vi "Imaign Pulse Control.vi"() -> ()   [LabVIEW 2012]
doc: "This VI is an example of how to use subVIs from the QC 9000 series driver to programmatically configure multiple channels and the system timer (To). This VI initializes the pulse generator, gets the number of channels in the unit, configures individual channel(s), configures the system timer (To), initiate pulse generation, and then closes communications with the pulse generator. By default the VI DOES NOT stop pulse generation when exiting!!! Not all trigger and gate features are supported by all models covered by this driver. Selection of an unsupported function will generate a software error and the command is not sent to the hardware.\n\n\nNotes:\n1) The pulse generator keypad is returned to \"Local\" mode when this VI terminates in order to restore manual control to the user.\n2) VISA Version 3.3 or higher must be installed to use this instrument driver."
uses:
  Examples/Support/Channel Parameters.ctl
  Examples/Support/System Parameters.ctl
  Quantum Composers 9000 Series.lvlib
panel:
  in  "VISA resource":refnum<visa-resource-name>="GPIB0::4::INSTR"
  in  "System Paramaters":T1={"Sys Period"=0.02, "Sys Mode"=enum."Single", "Sys Burst #"=0, "Sys DC On"=10, "Sys DC Off"=20, "Sys State"=TRUE, "Sys Gate"=TRUE, "Sys Trig Edge"=TRUE, "Sys Ext Mode"=enum."Triggered", "Sys Trig Lev"=2.0, "Sys Gate Lev "=2.5, "Sys Gate Mode"=enum."Disabled"} {"Sys Gate Lev" format="%.4p"; "Sys Trig Lev" format="%.4p"; "Sys Period" format="%.6p"}
  in  "Channel Parameters":T2[](array[typedef])=[{"Channel"=1, "Chan State"=TRUE, "Chan Sync Source"=0, "Chan Gate Logic"=enum."Disabled", "Chan Mode"=enum."Normal", "Chan Wait #"=0, "Chan Delay"=0.0, "Chan Width"=1e-05, "Chan Burst #"=0, "Chan DC On"=0, "Chan DC Off"=0, "Chan Polarity"=FALSE, "Chan MUX Value"=3, "Chan Level Out"=enum."TTL", "Chan Lev Adjust"=5.0, "Chan Gate Mode"=enum."Disabled"}, {"Channel"=2, "Chan State"=TRUE, "Chan Sync Source"=0, "Chan Gate Logic"=enum."Disabled", "Chan Mode"=enum."Normal", "Chan Wait #"=0, "Chan Delay"=0.0105, "Chan Width"=1e-05, "Chan Burst #"=0, "Chan DC On"=0, "Chan DC Off"=0, "Chan Polarity"=FALSE, "Chan MUX Value"=-1, "Chan Level Out"=enum."TTL", "Chan Lev Adjust"=0.0, "Chan Gate Mode"=enum."Disabled"}, {"Channel"=3, "Chan State"=TRUE, "Chan Sync Source"=0, "Chan Gate Logic"=enum."Disabled", "Chan Mode"=enum."Normal", "Chan Wait #"=30, "Chan Delay"=0.03, "Chan Width"=0.03, "Chan Burst #"=30, "Chan DC On"=30, "Chan DC Off"=30, "Chan Polarity"=FALSE, "Chan MUX Value"=-1, "Chan Level Out"=enum."TTL", "Chan Lev Adjust"=0.0, "Chan Gate Mode"=enum."Disabled"}, {"Channel"=4, "Chan State"=TRUE, "Chan Sync Source"=0, "Chan Gate Logic"=enum."Disabled", "Chan Mode"=enum."Normal", "Chan Wait #"=40, "Chan Delay"=0.04, "Chan Width"=0.04, "Chan Burst #"=40, "Chan DC On"=40, "Chan DC Off"=40, "Chan Polarity"=FALSE, "Chan MUX Value"=-1, "Chan Level Out"=enum."TTL", "Chan Lev Adjust"=0.0, "Chan Gate Mode"=enum."Disabled"}] {"Chan Sync Source" items=["System (To)", "Channel A", "Channel B", "Channel C", "Channel D", "Channel E", "Channel F", "Channel G", "Channel H"]; "Chan Width" format="%.3p"; "Chan Delay" format="%.3p"; "Chan MUX Value" min=-1 max=255; "Chan Lev Adjust" min=0.0 max=5.0 format="%.3p"; "Channel" items=["Channel A"=1, "Channel B"=2, "Channel C"=3, "Channel D"=4, "Channel E"=5, "Channel F"=6, "Channel G"=7, "Channel H"=8]}
  # "9000 Series\nPulse Generator\nExample Program"
  # "Notes:\n1.  The channel parameters \"Burst #\", \"DC On\", \"DC Off\", and \"Adjustable\" are only updated when operating in the corresponding mode.\n2.  The system parameters  \"Burst #\", \"DC On\", \"DC Off\", and \"Trig Level\"` are only updated when operating in the corresponding mode."
  # "Input"
  # "Triggered"
  # "Gated"
  # "Mode"
  # "Burst"
  # "Duty\nCycle"
  # "Input"
  # "Normal\nSingle\nBurst"
  # "Burst"
  # "Duty Cycle"
  # "Output"
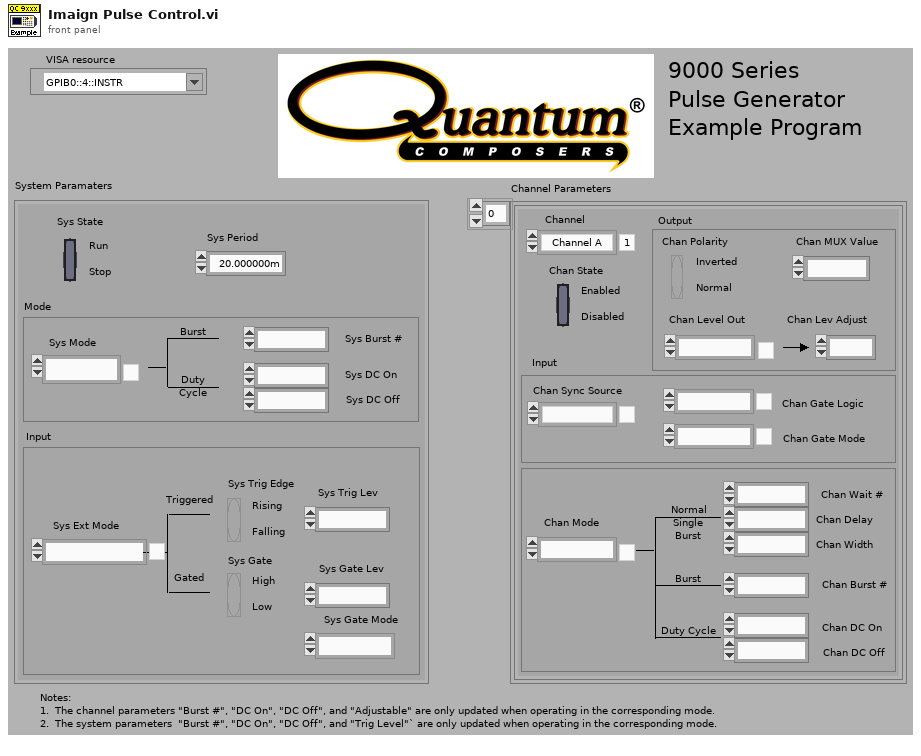
[diagram p1: front panel]
types:
  T1 = typedef "System Parameters.ctl" = cluster{"Sys Period":dbl, "Sys Mode":enum16{"Normal", "Single", "Burst", "Duty Cycle"}, "Sys Burst #":i32, "Sys DC On":i32, "Sys DC Off":i32, "Sys State":bool, "Sys Gate":bool, "Sys Trig Edge":bool, "Sys Ext Mode":enum16{"Disabled", "Triggered", "Gated", "Triggered & Gated"}, "Sys Trig Lev":dbl, "Sys Gate Lev ":dbl, "Sys Gate Mode":enum16{"Disabled", "Pulse Inhibit", "Output Inhibit", "Channel"}}
  T2 = typedef "Channel Parameters.ctl" = cluster{"Channel":i32, "Chan State":bool, "Chan Sync Source":i32, "Chan Gate Logic":enum16{"Disabled", "Low", "High"}, "Chan Mode":enum16{"Normal", "Single", "Burst", "Duty Cycle"}, "Chan Wait #":i32, "Chan Delay":dbl, "Chan Width":dbl, "Chan Burst #":i32, "Chan DC On":i32, "Chan DC Off":i32, "Chan Polarity":bool, "Chan MUX Value":i32, "Chan Level Out":enum16{"TTL", "Adjustable", "35 Volt", "Optical"}, "Chan Lev Adjust":dbl, "Chan Gate Mode":enum16{"Disabled", "Pulse Inhibit", "Output Inhibit"}}
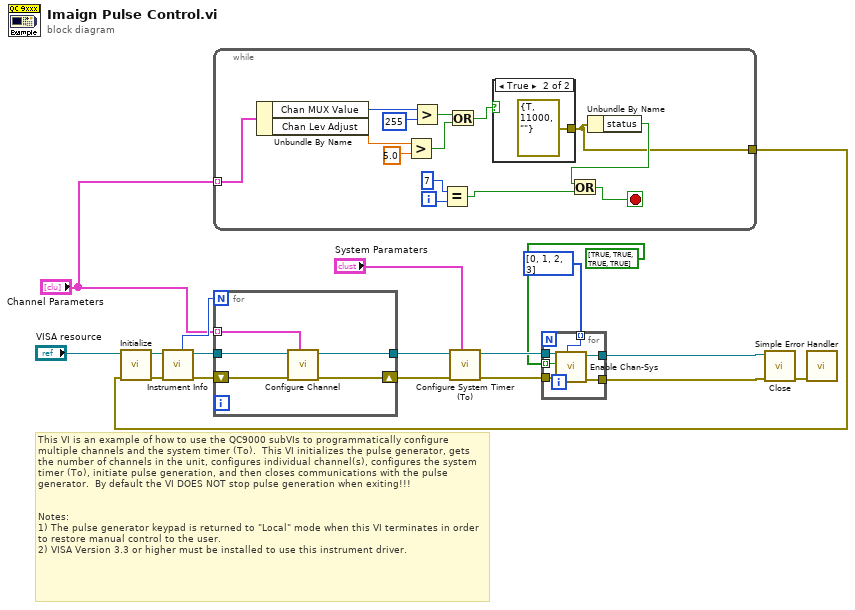
[diagram p0: block diagram]
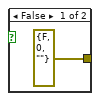
[diagram p2: hidden frame]
diagram:
  # "This VI is an example of how to use the QC9000 subVIs to programmatically configure multiple channels and the system timer (To).  This VI initializes the pulse generator, gets the number of channels in the unit, configures individual channel(s), configures the system timer (To), initiate pulse generation, and then closes communications with the pulse generator.  By default the VI DOES NOT stop pulse generation when exiting!!!\n\n\nNotes:\n1) The pulse generator keypad is returned to \"Local\" mode when this VI terminates in order to restore manual control to the user.\n2) VISA Version 3.3 or higher must be installed to use this instrument driver."
  n1 = while {
    tunnel: "Channel Parameters" -> [w32] mode=indexing
    tunnel: [w19] -> w4
    i -> [w30]
    stop <- w20 stop-if-true
    n2 = Unbundle By Name(w32) -> ("Chan MUX Value"=w25:i32, "Chan Lev Adjust"=w28:dbl)
    n3 = Greater?(x=w28, y=5.0) -> (0:w26:bool)
    n4 = Greater?(x=w25, y=255) -> (0:w23:bool)
    n5 = Equal?(x=7, y=w30) -> (x = y?=w22:bool)
    n6 = Or(x=w23, y=w26) -> (x .or. y?=w27:bool)
    n7 = case shown="True" w27 {
      tunnel: [errorcluster {"status"=FALSE, "code"=0, "source"=""} ("error constant") errorcluster {"status"=TRUE, "code"=11000, "source"=""} ("error constant")] -> w19
      frame False {
      }
      frame True {
      }
    }
    n8 = Unbundle By Name(w19) -> ("status"=w21:bool)
    n9 = Or(x=w21, y=w22) -> (x .or. y?=w20:bool)
  }
  n10 = call "Initialize.vi"("error in (no error)"=w4, "VISA resource name"="VISA resource") -> ("error out"=w14:errorcluster, "VISA resource name out"=w15:refnum<visa-resource-name>)  [unwired: 8 in]
  n11 = call "Instrument Info.vi"("error in (no error)"=w14, "VISA resource name"=w15) -> ("error out"=w12:errorcluster, "VISA resource name out"=w16:refnum<visa-resource-name>, "Channels"=w11:i32)  [unwired: 6 in, 1 out]
  n12 = for {
    N: w11 -> [_]
    tunnel: [w39] -> w18
    tunnel: "Channel Parameters" -> [w38] mode=indexing
    tunnel: w16 -> [w37]
    shift-right: [w36] -> w13
    shift-left: w12 -> [w35]
    n13 = call "Configure Channel.vi"("Chan Parameters"=w38, "error in (no error)"=w35, "VISA resource name"=w37) -> ("error out"=w36:errorcluster, "VISA resource name out"=w39:refnum<visa-resource-name>)  [unwired: 7 in]
  }
  n14 = call "Configure System Timer (To).vi"("System Parameters"="System Paramaters", "error in (no error)"=w13, "VISA resource name"=w18) -> ("error out"=w7:errorcluster, "VISA resource name out"=w8:refnum<visa-resource-name>)  [unwired: 7 in]
  n15 = for {
    tunnel: w8 -> [w45]
    tunnel: w7 -> [w44]
    tunnel: [w43] -> w6
    tunnel: [w42] -> w5
    tunnel: i32[] [0, 1, 2, 3] -> [w41] mode=indexing
    tunnel: bool[] [TRUE, TRUE, TRUE, TRUE] -> [w40] mode=indexing
    n16 = call "Enable Chan-Sys.vi"("Channel (1:Chan A)"=w41, "error in (no error)"=w44, "State (T:Enabled)"=w40, "VISA resource name"=w45) -> ("error out"=w42:errorcluster, "VISA resource name out"=w43:refnum<visa-resource-name>)  [unwired: 6 in]
  }
  n17 = call "Close.vi"("error in (no error)"=w5, "VISA resource name"=w6) -> ("error out"=w10:errorcluster)  [unwired: 9 in]
  n18 = call <vilib>:"Simple Error Handler.vi"("error in (no error)"=w10) -> ()  [unwired: 4 in, 5 out]
